vi "Main.vi"(8 "error in":errorcluster, 11 "Head Worker in":refnum<class "Head Worker.lvclass">) -> (0 "error out":errorcluster, 3 "Head Worker out":refnum<class "Head Worker.lvclass">)   [LabVIEW 2023, in "Head Worker.lvclass"]
doc: "The <b>Queued Message Handler</b> of the Worker that owns this VI."
uses:
  Head Worker.lvclass
  C:/Program Files (x86)/National Instruments/LabVIEW 2023/vi.lib/addons/_Workers/Library/Classes/Worker/Worker.lvclass
  Generated_server/RPC Service/streamai/typeDefs/Server gRPC UEs.ctl
  <vilib>/gRPC/LabVIEW gRPC Library/Server API/typeDefs/gRPCId Cluster.ctl
  <vilib>/gRPC/LabVIEW gRPC Library/Shared/grpcId.ctl
  Head Worker.lvclass/Head Worker.ctl
  Generated_server/RPC Service/streamai/streamai.lvclass
  Generated_server/RPC Service/streamai/streamai.lvclass/streamai.ctl
  rql_Start Acquisition.ctl
  rql_Stop Acquisition.ctl
  Generated_server/RPC Messages/google_protobuf_Empty.ctl
  Analog Signal/rqp_Set Signal Config.ctl
  Analog Signal/Support/Signal Config.ctl
  Analog Signal/Support/Signal Type.ctl
  Analog Signal/rqp_Set Sampling.ctl
  Analog Signal/Support/Sampling Config.ctl
  Initialization Data.ctl
  Response Cases.ctl
  <vilib>/gRPC/LabVIEW gRPC Servicer/Servicer/Servicer.lvclass
  <vilib>/gRPC/LabVIEW gRPC Servicer/ServiceBase/ServiceBase.lvclass
  Analog Signal/rqp_Insert to Subpanel.ctl
  Generated_server/RPC Messages/streamai_status.ctl
  Generated_server/RPC Messages/streamai_waveform.ctl
  Generated_server/RPC Messages/google_protobuf_Timestamp.ctl
  <vilib>/addons/_Workers/Library/Classes/Message Queue/Message Queue.lvclass
  Analog Signal/Analog Signal.lvclass
  Generated_server/Generated_server.lvlib
  <vilib>/gRPC/LabVIEW gRPC Library/grpc-lvsupport-release.lvlib
  C:/Program Files (x86)/National Instruments/LabVIEW 2023/vi.lib/addons/_Workers/Library/Classes/Workers Object/Workers Object.lvclass
  C:/Users/Admin/Documents/Learn/LabVIEW/Github_Repo/LabVIEW-Worker-gRPC/Worker gRPC Server/Workers/Head Worker/Head Worker.lvclass
panel:
  in  "Acq Status":bool
  in  "Start AI":bool
  out "Status":string
  out "Listening Port":i32
  in  "Server Address":string="localhost:50051"
  in  "Start Button":bool
  # "gRPC Server"
  # "Debug"
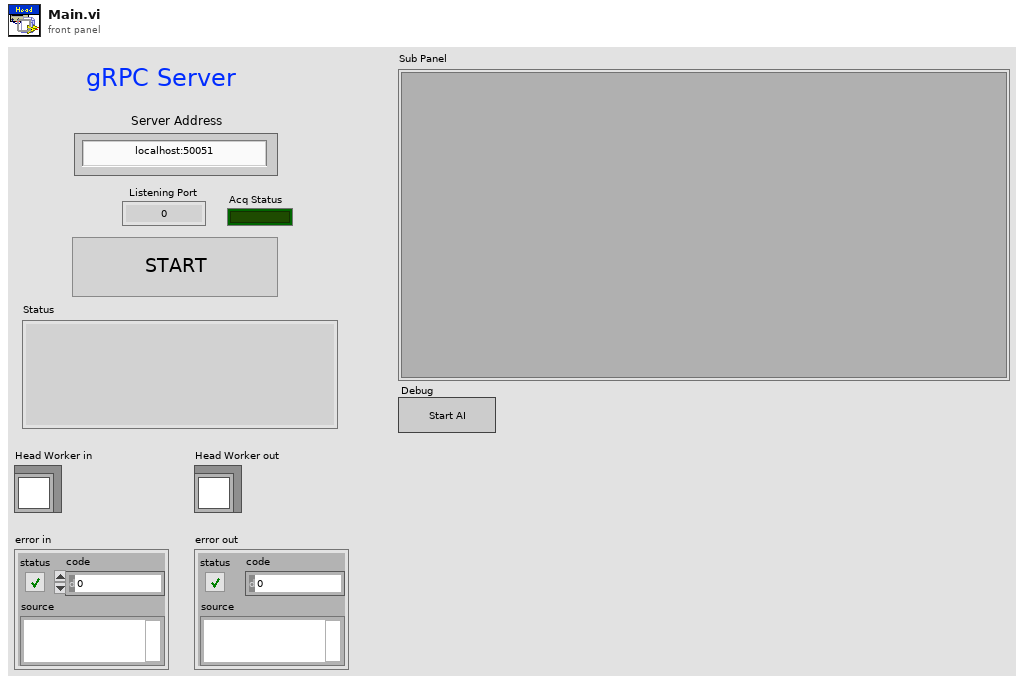
[diagram p1: front panel]
types:
  T1 = typedef "Generated_server.lvlib/streamai.lvclass/Server gRPC UEs.ctl" = cluster{"streamai startacq gRPC UE":refnum<user-event>, "streamai stopacq gRPC UE":refnum<user-event>, "streamai setSignalConfig gRPC UE":refnum<user-event>, "streamai setSamplingConfig gRPC UE":refnum<user-event>}
  T2 = typedef "Head Worker.lvclass/Event Data.ctl" = cluster{"gRPC streamAI services":refnum<user-event>, "gRPC Server Stop":refnum<user-event>}
  T3 = enum32{"Invalid", "Standard", "Closed", "Hidden", "Minimized", "Maximized"}
  T4 = typedef "Head Worker.lvclass/Initialization Data.ctl" = cluster{"Response Cases":T5}
  T5 = typedef "Head Worker.lvclass/Response Cases.ctl" = cluster{"gRPC server":refnum<class "Servicer.lvclass">, "gRPC streamAI":refnum<class "ServiceBase.lvclass">, "gRPCid Startacq":T6}
  T6 = typedef "grpc-lvsupport-release.lvlib/grpcId.ctl" = u64
  T7 = typedef "Analog Signal.lvclass/rqp_Insert to Subpanel.ctl" = cluster{"Sub Panel Ref":refnum<vi>}
  T8 = typedef "Head Worker.lvclass/rql_Start Acquisition.ctl" = cluster{"gRPCid Startacq":T6}
  T9 = typedef "Generated_server.lvlib/streamai_status.ctl" = cluster{"acquisition":bool}
  T10 = typedef "Head Worker.lvclass/rql_Stop Acquisition.ctl" = cluster{"gRPCid Stopacq":T6}
  T11 = typedef "Generated_server.lvlib/streamai_waveform.ctl" = cluster{"t0":T12, "delta_t":dbl, "values":dbl[]}
  T12 = typedef "Generated_server.lvlib/google_protobuf_Timestamp.ctl" = cluster{"seconds":i64, "nanos":i32}
  T13 = typedef "Generated_server.lvlib/google_protobuf_Empty.ctl" = cluster{"void":string}
  T14 = typedef "Analog Signal.lvclass/Signal Type.ctl" = enum16{"Sine Wave", "Square Wave"}
  T15 = typedef "Analog Signal.lvclass/rqp_Set Sampling.ctl" = cluster{"Sampling_Config":T16}
  T16 = typedef "Analog Signal.lvclass/Sampling Config.ctl" = cluster{"Fs":dbl, "#s":dbl}
  T17 = typedef "Analog Signal.lvclass/rsp_Acquisition.ctl" = cluster{"Waveform":waveform(dbl)}
  T18 = typedef "Analog Signal.lvclass/rqp_Set Signal Config.ctl" = cluster{"Signal_Config":T19, "Signal Type":T14}
  T19 = typedef "Analog Signal.lvclass/Signal Config.ctl" = cluster{"offset":dbl, "frequency":dbl, "amplitude":dbl}
  T20 = typedef "Generated_server.lvlib/streamai_signalConfig.ctl" = cluster{"type":T21, "offset":dbl, "frequency":dbl, "amplitude":dbl}
  T21 = typedef "Generated_server.lvlib/streamai_SignalType.ctl" = enum32{"SIGNAL_SINE", "SIGNAL_SQUARE"}
  T22 = typedef "Generated_server.lvlib/streamai_samplingConfig.ctl" = cluster{"sample_rate":dbl, "num_sample":i32}
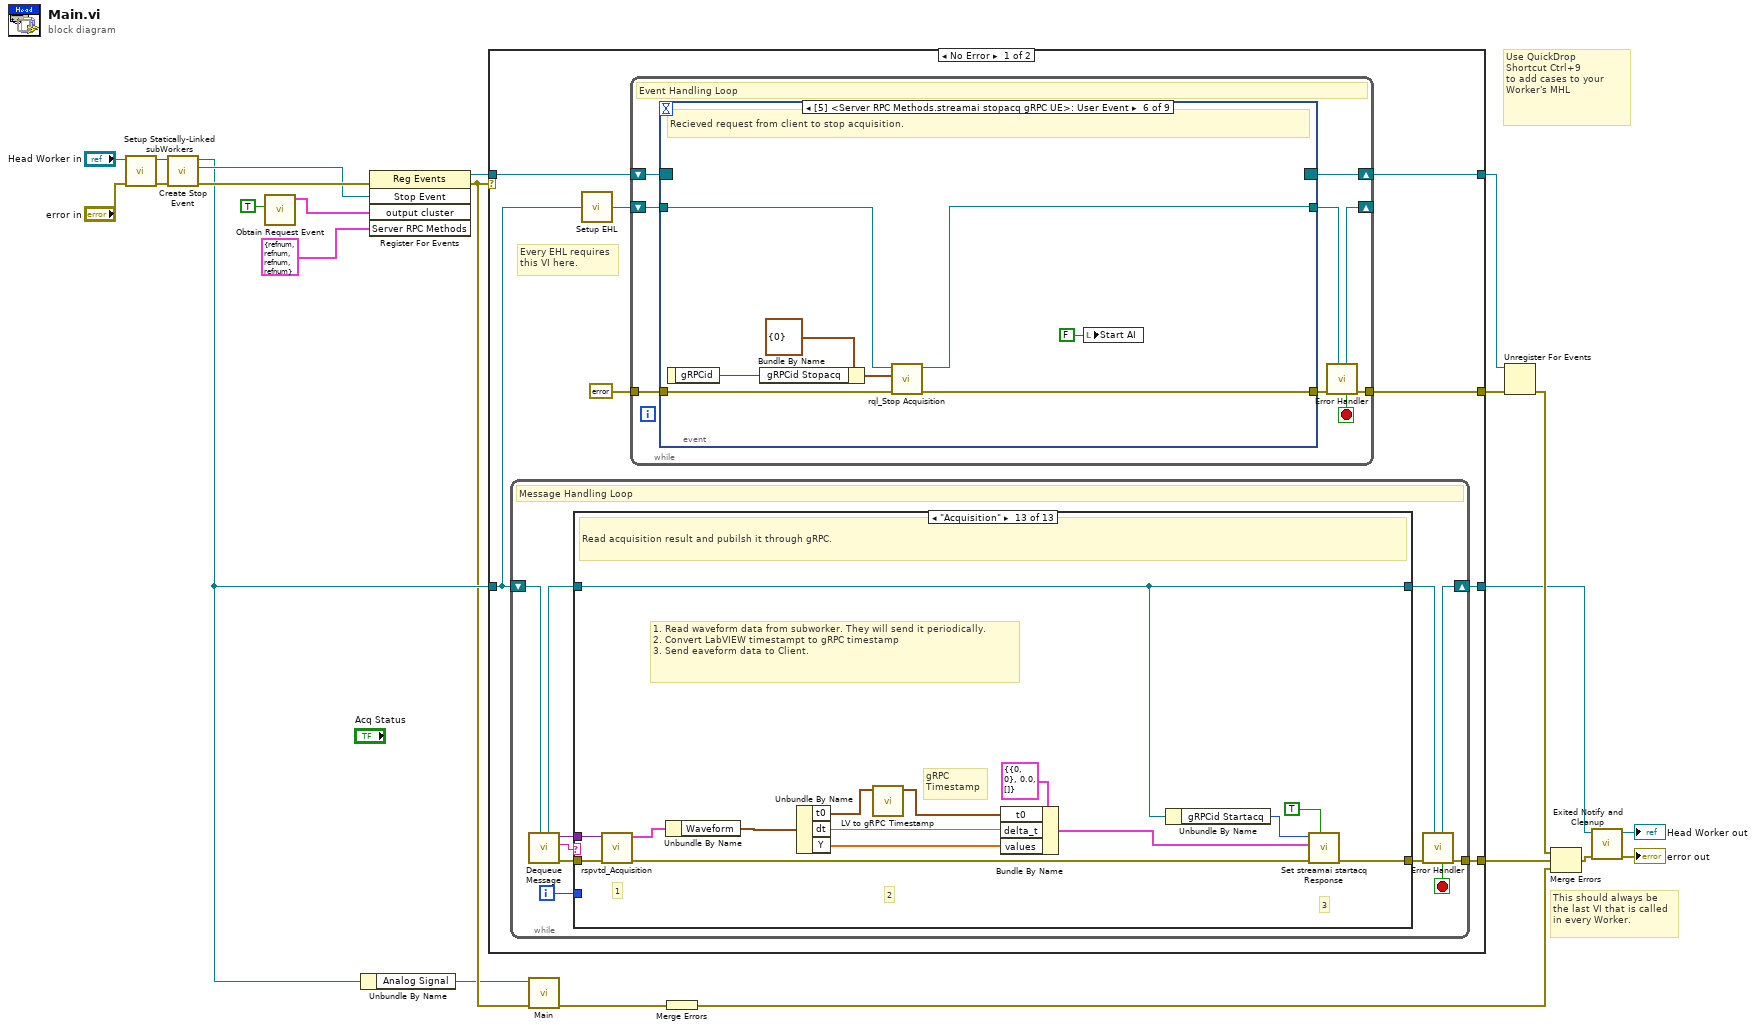
[diagram p0: block diagram]
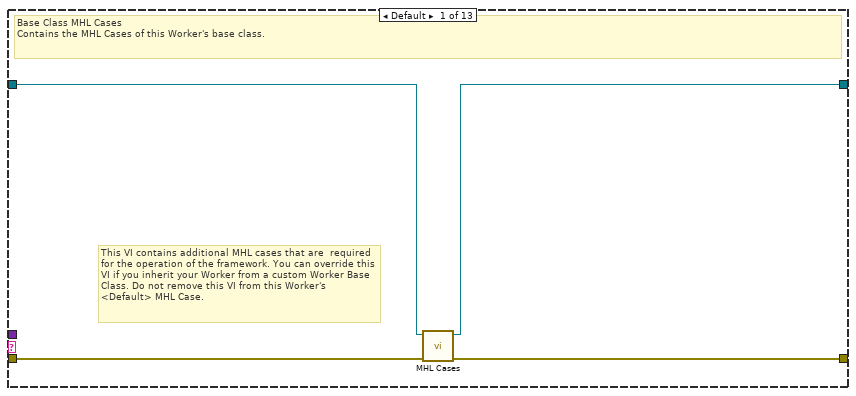
[diagram p2: hidden frame]
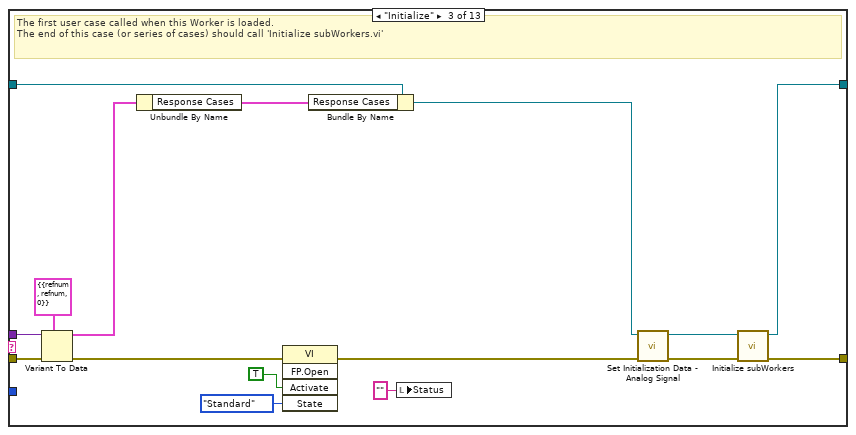
[diagram p4: hidden frame]
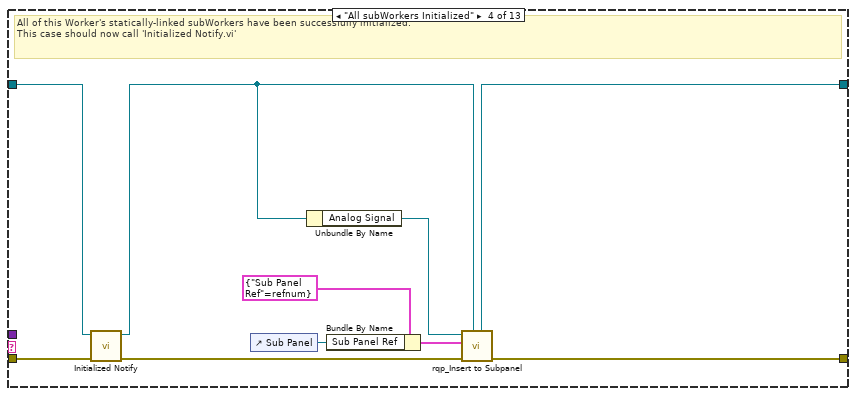
[diagram p5: hidden frame]
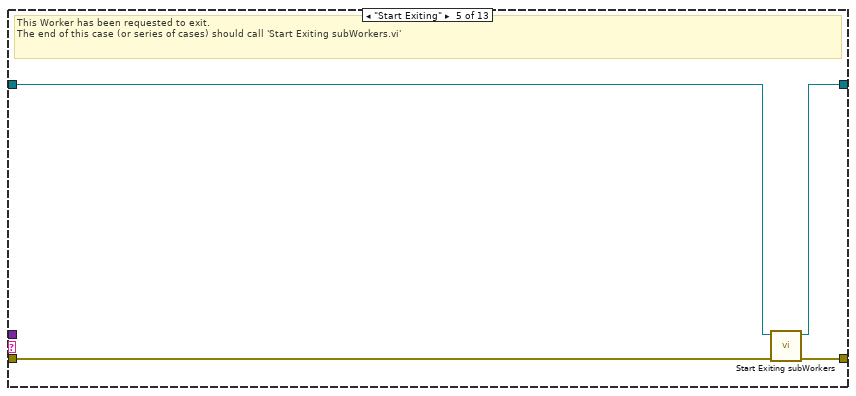
[diagram p6: hidden frame]
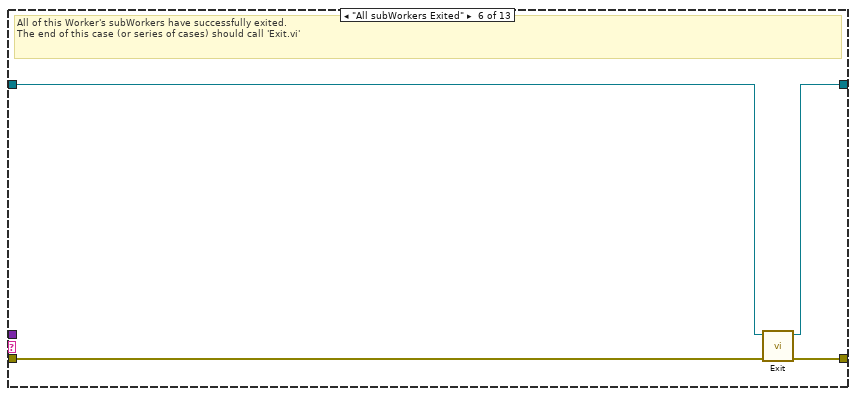
[diagram p7: hidden frame]
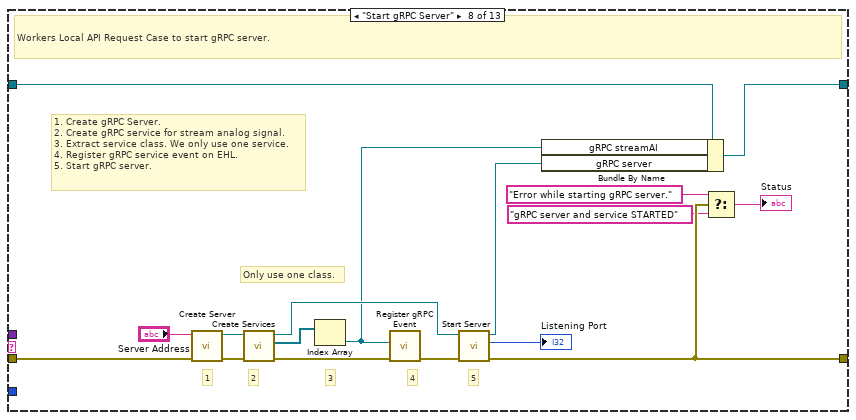
[diagram p9: hidden frame]
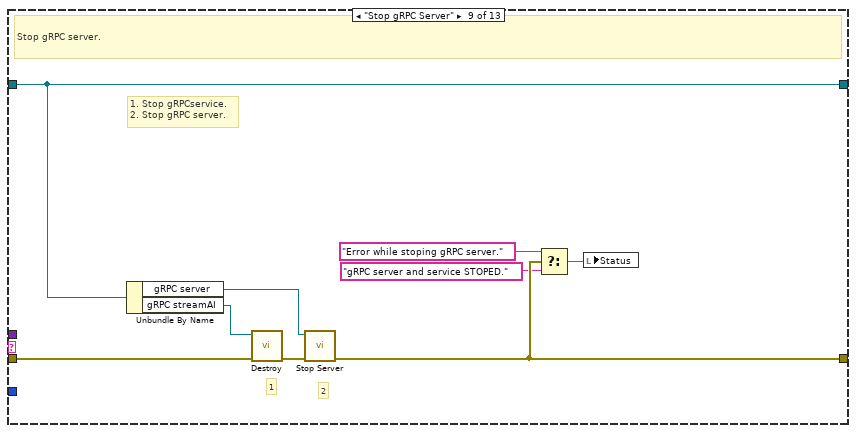
[diagram p10: hidden frame]
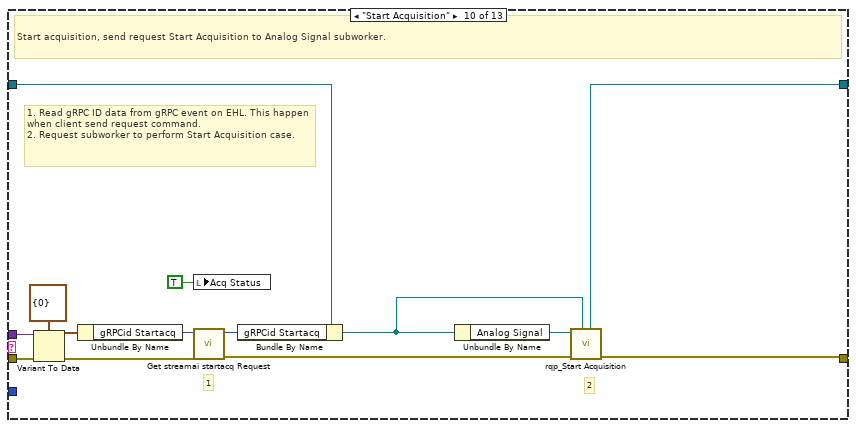
[diagram p11: hidden frame]
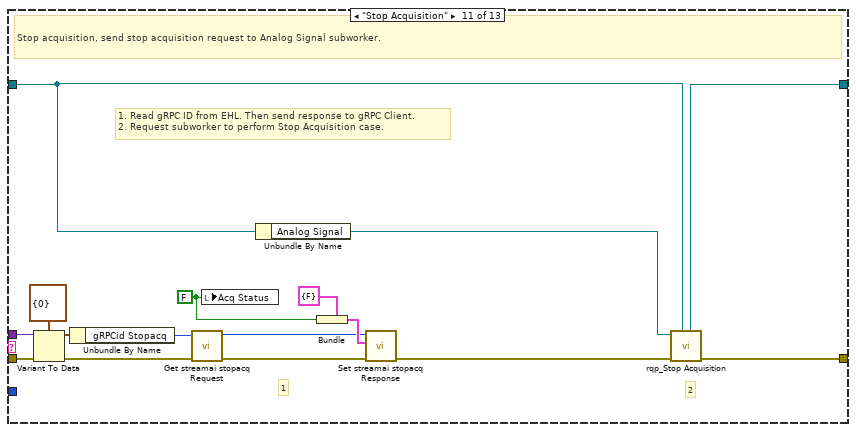
[diagram p12: hidden frame]
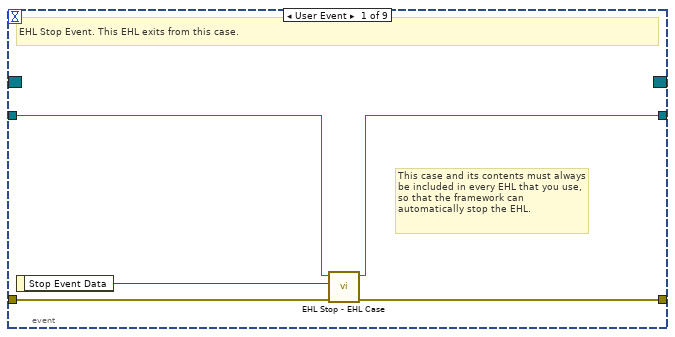
[diagram p14: hidden frame]
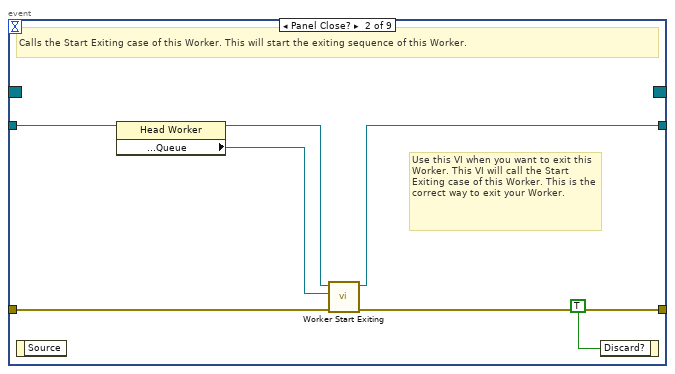
[diagram p15: hidden frame]
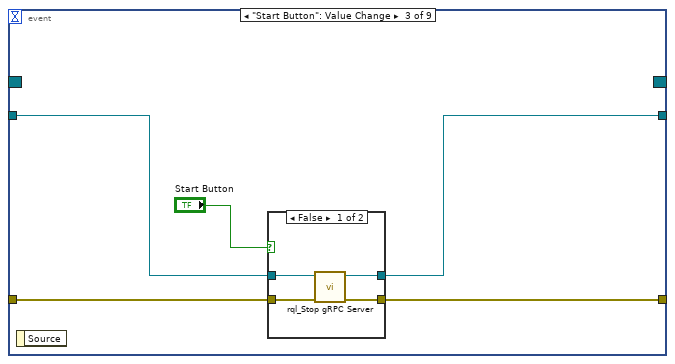
[diagram p16: hidden frame]
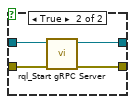
[diagram p17: hidden frame]
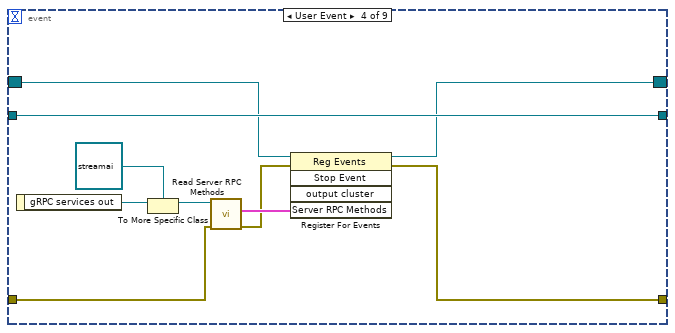
[diagram p18: hidden frame]
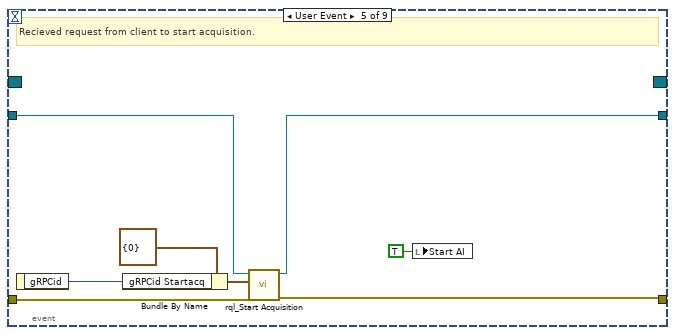
[diagram p19: hidden frame]
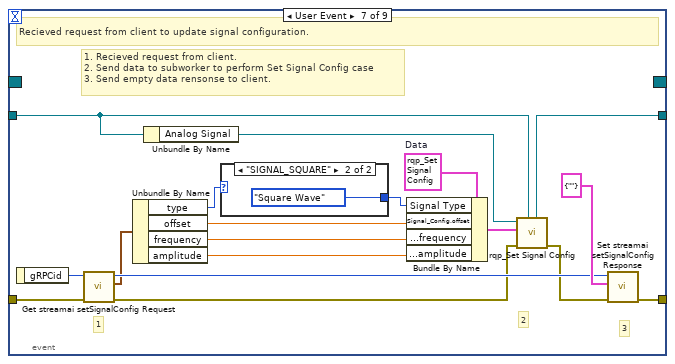
[diagram p20: hidden frame]
diagram:
  # "Use QuickDrop\nShortcut Ctrl+9\nto add cases to your\nWorker's MHL"
  # "This should always be the last VI that is called in every Worker."
  n1 = call "Setup Statically-Linked subWorkers.vi"("error in"="error in", "Head Worker in"="Head Worker in") -> ("error out"=w9:errorcluster, "Head Worker out"=w7:refnum<class "Head Worker.lvclass">)  [unwired: 8 in]
  n2 = call-dynamic "Create Stop Event.vi"("error in"=w9, "Worker"=w7) -> ("error out"=w18:errorcluster, "Stop Event"=w15:refnum<user-event>, "Worker out"=w12:refnum<class "Head Worker.lvclass">)  [unwired: 7 in]
  n3 = call "Obtain Request Event.vi"("Create New"=TRUE) -> ("output cluster"=w3:T2)  [unwired: 9 in, 1 out]
  n4 = Unbundle By Name(w12) -> ("Analog Signal"=w4:refnum<class "Analog Signal.lvclass">)
  n5 = register-events(error in=w18, w15, w3, T1 {"streamai startacq gRPC UE"=refnum, "streamai stopacq gRPC UE"=refnum, "streamai setSignalConfig gRPC UE"=refnum, "streamai setSamplingConfig gRPC UE"=refnum} ("Server RPC Methods")) -> (reference out=w17:refnum<event-registration>, error out=w10:errorcluster)  [unwired: 1 in]
  n6 = case shown="No Error" w10 {
    tunnel: w12 -> [w26 w268]
    tunnel: [w24 w269] -> w16
    tunnel: w17 -> [w31 w270]
    tunnel: [w28 w271] -> w22
    tunnel: [w30 w270] -> w21
    tunnel: [w25 w267] -> w19
    selector: w10 -> [_ w271]
    frame No Error {
      # "Every EHL requires\nthis VI here."
      n7 = while {
        shift-right: [w40] -> w25
        shift-left: w26 -> [w42]
        tunnel: [w41] -> w24
        i -> [w33]
        stop <- w34 stop-if-true
        # "Message Handling Loop"
        n8 = call-dynamic "Dequeue Message.vi"("Worker"=w42) -> ("error out"=w39:errorcluster, "Case out"=w35:string, "Data out"=w32:variant, "Worker out"=w37:refnum<class "Head Worker.lvclass">)  [unwired: 6 in, 1 out]
        n9 = case "Worker MHL Case Structure (DO NOT CHANGE LABEL NAME)" shown="\"Acquisition\"" w35 {
          tunnel: w39 -> [w46 w47 w62 w73 w75 w82 w84 w101 w110 w124 w140 w142 w157]
          tunnel: [w45 w47 w64 w71 w78 w81 w84 w98 w109 w116 w129 w142 w153] -> w38
          tunnel: w37 -> [w44 w48 w61 w74 w76 w80 w83 w100 w108 w115 w136 w141 w152]
          tunnel: [w43 w48 w63 w65 w77 w79 w83 w99 w108 w114 w135 w141 w152] -> w36
          tunnel: w33 -> [_ _ _ _ _ _ _ _ _ _ _ _ _]
          tunnel: w32 -> [_ _ w60 _ _ _ _ _ _ w122 w138 _ w155]
          frame Default {
            # "This VI contains additional MHL cases that are  required for the operation of the framework. You can override this VI if you inherit your Worker from a custom Worker Base Class. Do not remove this VI from this Worker's <Default> MHL Case."
            # "Base Class MHL Cases\nContains the MHL Cases of this Worker's base class."
            n10 = call-dynamic "MHL Cases.vi"("error in"=w46, "Worker in"=w44) -> ("error out"=w45:errorcluster, "Worker out"=w43:refnum<class "Head Worker.lvclass">)  [unwired: 8 in]
          }
          frame "------------ FRAMEWORK CASES -----------" {
            # "Start of Workers Framework Cases"
          }
          frame "Initialize" {
            # "The first user case called when this Worker is loaded.\nThe end of this case (or series of cases) should call 'Initialize subWorkers.vi'"
            n11 = Variant To Data(error in=w62, type=T4 {"Response Cases"={"gRPC server"=refnum, "gRPC streamAI"=refnum, "gRPCid Startacq"=0}} ("Initialization Data"), Variant=w60) -> (data=w59:T4, error out=w55:errorcluster)
            n12 = Unbundle By Name(w59) -> ("Response Cases"=w58:T5)
            n13 = invoke class="VI" method="FP.Open"(error in=w55, "Activate"=TRUE ("Activate?"), "State"=T3."Standard") -> (error out=w54:errorcluster)  [unwired: 2 in, 4 out]
            n14 = Bundle By Name(cluster=w61, "Response Cases"=w58) -> (w56:refnum<class "Head Worker.lvclass">)
            n15 = local write "Status"("" ("Status")) -> ()
            n16 = call "Set Initialization Data - Analog Signal.vi"("error in"=w54, "Head Worker in"=w56) -> ("error out"=w50:errorcluster, "Head Worker out"=w51:refnum<class "Head Worker.lvclass">)  [unwired: 8 in]
            n17 = call-dynamic "Initialize subWorkers.vi"("error in"=w50, "Worker"=w51) -> ("error out"=w64:errorcluster, "dup Worker out"=w63:refnum<class "Head Worker.lvclass">)  [unwired: 8 in]
          }
          frame "All subWorkers Initialized" {
            # "All of this Worker's statically-linked subWorkers have been successfully initialized.\nThis case should now call 'Initialized Notify.vi'"
            n18 = call-dynamic "Initialized Notify.vi"("error in"=w73, "Worker"=w74) -> ("error out"=w72:errorcluster, "dup Worker out"=w66:refnum<class "Head Worker.lvclass">)  [unwired: 8 in]
            n19 = control-ref of="Sub Panel"() -> (w70:refnum<vi>)
            n20 = Unbundle By Name(w66) -> ("Analog Signal"=w67:refnum<class "Analog Signal.lvclass">)
            n21 = Bundle By Name(cluster=T7 {"Sub Panel Ref"=refnum} ("Data in"), "Sub Panel Ref"=w70) -> (w68:T7)
            n22 = call "rqp_Insert to Subpanel.vi"("Caller in"=w66, "error in"=w72, "Data in"=w68, "Analog Signal in"=w67) -> ("error out"=w71:errorcluster, "dup Caller out"=w65:refnum<class "Head Worker.lvclass">)  [unwired: 5 in, 1 out]
          }
          frame "Start Exiting" {
            # "This Worker has been requested to exit. \nThe end of this case (or series of cases) should call 'Start Exiting subWorkers.vi'"
            n23 = call-dynamic "Start Exiting subWorkers.vi"("error_in"=w75, "Worker"=w76) -> ("error out"=w78:errorcluster, "dup Worker out"=w77:refnum<class "Head Worker.lvclass">)  [unwired: 8 in]
          }
          frame "All subWorkers Exited" {
            # "All of this Worker's subWorkers have successfully exited. \nThe end of this case (or series of cases) should call 'Exit.vi'"
            n24 = call-dynamic "Exit.vi"("error_in"=w82, "Worker"=w80) -> ("error out"=w81:errorcluster, "dup Worker out"=w79:refnum<class "Head Worker.lvclass">)  [unwired: 8 in]
          }
          frame "------------- LOCAL API CASES -------------" {
            # "Start of Workers Local API Cases"
          }
          frame "Start gRPC Server" {
            # "1. Create gRPC Server.\n2. Create gRPC service for stream analog signal.\n3. Extract service class. We only use one service.\n4. Register gRPC service event on EHL.\n5. Start gRPC server."
            # "5"
            # "4"
            # "3"
            # "2"
            # "1"
            # "Only use one class."
            # "Workers Local API Request Case to start gRPC server."
            n25 = call <vilib>:"Create Server.vi"("error in"=w101, "Server Address"="Server Address") -> ("error out"=w97:errorcluster, "gRPC server out"=w96:refnum<class "Servicer.lvclass">)  [unwired: 8 in]
            n26 = call "Create Services.vi"("error in (no error)"=w97, "gRPC server in"=w96) -> ("error out"=w87:errorcluster, "gRPC services out"=w88:refnum<class "ServiceBase.lvclass">[], "gRPC server out"=w94:refnum<class "Servicer.lvclass">)  [unwired: 7 in]
            n27 = Index Array(array=w88) -> (element=w85:refnum<class "ServiceBase.lvclass">)  [unwired: 1 in]
            n28 = call "Register gRPC Event.vi"("error in (no error)"=w87, "Event Data"=w85) -> ("error out"=w86:errorcluster)  [unwired: 9 in]
            n29 = call <vilib>:"Start Server.vi"("error in"=w86, "gRPC server in"=w94) -> ("error out"=w98:errorcluster, "Listening Port"=→"Listening Port":i32, "gRPC server out"=w92:refnum<class "Servicer.lvclass">)  [unwired: 7 in]
            n30 = Bundle By Name(cluster=w100, "gRPC streamAI"=w85, "gRPC server"=w92) -> (w99:refnum<class "Head Worker.lvclass">)
            n31 = Select(t="Error while starting gRPC server.", s=w98, f="gRPC server and service STARTED") -> (s? t:f=→"Status":string)
          }
          frame "Stop gRPC Server" {
            # "1. Stop gRPCservice.\n2. Stop gRPC server."
            # "2"
            # "1"
            # "Stop gRPC server."
            n32 = Unbundle By Name(w108) -> ("gRPC server"=w105:refnum<class "Servicer.lvclass">, "gRPC streamAI"=w107:refnum<class "ServiceBase.lvclass">)
            n33 = call-dynamic "Destroy.vi"("error in"=w110, "gRPC service in"=w107) -> ("error out"=w106:errorcluster)  [unwired: 8 in, 1 out]
            n34 = call <vilib>:"Stop Server.vi"("error in"=w106, "gRPC server in"=w105) -> ("error out"=w109:errorcluster)  [unwired: 9 in]
            n35 = Select(t="Error while stoping gRPC server.", s=w109, f="gRPC server and service STOPED.") -> (s? t:f=w102:string)
            n36 = local write "Status"(w102) -> ()
          }
          frame "Start Acquisition" {
            # "1. Read gRPC ID data from gRPC event on EHL. This happen when client send request command.\n2. Request subworker to perform Start Acquisition case."
            # "2"
            # "1"
            # "Start acquisition, send request Start Acquisition to Analog Signal subworker."
            n37 = Variant To Data(error in=w124, type=T8 {"gRPCid Startacq"=0} ("Data"), Variant=w122) -> (data=w121:T8, error out=w118:errorcluster)
            n38 = Unbundle By Name(w121) -> ("gRPCid Startacq"=w120:T6)
            n39 = local write "Acq Status"(TRUE ("Acq Status?")) -> ()
            n40 = call "Get streamai startacq Request.vi"("error in (no error)"=w118, "gRPCid"=w120) -> ("error out"=w117:errorcluster, "gRPCid out"=w112:T6)  [unwired: 7 in, 1 out]
            n41 = Bundle By Name(cluster=w115, "gRPCid Startacq"=w112) -> (w113:refnum<class "Head Worker.lvclass">)
            n42 = Unbundle By Name(w113) -> ("Analog Signal"=w119:refnum<class "Analog Signal.lvclass">)
            n43 = call "rqp_Start Acquisition.vi"("Caller in"=w113, "error in"=w117, "Analog Signal in"=w119) -> ("error out"=w116:errorcluster, "dup Caller out"=w114:refnum<class "Head Worker.lvclass">)  [unwired: 6 in, 1 out]
          }
          frame "Stop Acquisition" {
            w125 = FALSE ("Acq Status")
            # "1. Read gRPC ID from EHL. Then send response to gRPC Client.\n2. Request subworker to perform Stop Acquisition case."
            # "2"
            # "1"
            # "Stop acquisition, send stop acquisition request to Analog Signal subworker."
            n44 = Variant To Data(error in=w140, type=T10 {"gRPCid Stopacq"=0} ("Data"), Variant=w138) -> (data=w128:T10, error out=w131:errorcluster)
            n45 = Unbundle By Name(w128) -> ("gRPCid Stopacq"=w127:T6)
            n46 = call "Get streamai stopacq Request.vi"("error in (no error)"=w131, "gRPCid"=w127) -> ("error out"=w130:errorcluster, "gRPCid out"=w133:T6)  [unwired: 7 in, 1 out]
            n47 = local write "Acq Status"(w125) -> ()
            n48 = Unbundle By Name(w136) -> ("Analog Signal"=w137:refnum<class "Analog Signal.lvclass">)
            n49 = Bundle(cluster=T9 {"acquisition"=FALSE} ("Message Data"), "acquisition"=w125) -> (w134:T9)
            n50 = call "Set streamai stopacq Response.vi"("error in (no error)"=w130, "Message Data"=w134, "gRPCid in"=w133) -> ("error out"=w126:errorcluster)  [unwired: 8 in]
            n51 = call "rqp_Stop Acquisition.vi"("Caller in"=w136, "error in"=w126, "Analog Signal in"=w137) -> ("error out"=w129:errorcluster, "dup Caller out"=w135:refnum<class "Head Worker.lvclass">)  [unwired: 6 in, 1 out]
          }
          frame "------------- RESPONSE CASES --------------" {
            # "Start of Workers Response Cases"
          }
          frame "Acquisition" {
            # "3"
            # "2"
            # "1"
            # "1. Read waveform data from subworker. They will send it periodically.\n2. Convert LabVIEW timestampt to gRPC timestamp\n3. Send eaveform data to Client."
            # "gRPC\nTimestamp"
            # "Read acquisition result and pubilsh it through gRPC."
            n52 = call "rspvtd_Acquisition.vi"("error in"=w157, "Data in"=w155) -> ("error out"=w156:errorcluster, "Data out"=w154:T17)  [unwired: 8 in]
            n53 = Unbundle By Name(w154) -> ("Waveform"=w148:waveform(dbl))
            n54 = Unbundle By Name(w148) -> ("t0"=w144:timestamp, "dt"=w146:dbl, "Y"=w147:dbl[])
            n55 = call "LV to gRPC Timestamp.vi"("LV Timestamp"=w144) -> ("gRPC Timestamp"=w143:T12)  [unwired: 10 in]
            n56 = Bundle By Name(cluster=T11 {"t0"={"seconds"=0, "nanos"=0}, "delta_t"=0.0, "values"=[]} ("Message Data"), "t0"=w143, "delta_t"=w146, "values"=w147) -> (w145:T11)
            n57 = Unbundle By Name(w152) -> ("gRPCid Startacq"=w151:T6)
            n58 = call "Set streamai startacq Response.vi"("Streaming? (F)"=TRUE, "error in (no error)"=w156, "Message Data"=w145, "gRPCid in"=w151) -> ("error out"=w153:errorcluster)  [unwired: 7 in]
          }
        }
        n59 = call-dynamic "Error Handler.vi"("Worker"=w36, "error_in"=w38) -> ("error out"=w41:errorcluster, "Stop Loop"=w34:bool, "Worker out"=w40:refnum<class "Head Worker.lvclass">)  [unwired: 7 in]
      }
      n60 = call-dynamic "Setup EHL.vi"("Worker"=w26) -> ("Worker out"=w27:refnum<class "Head Worker.lvclass">)  [unwired: 14 in]
      n61 = while "Event Handling Loop" {
        shift-right: [w166] -> w30
        shift-left: w31 -> [w165]
        tunnel: [w161] -> w28
        tunnel: errorcluster {"status"=FALSE, "code"=0, "source"=""} ("error constant") -> [w163]
        shift-right: [w159] -> _
        shift-left: w27 -> [w164]
        stop <- w158 stop-if-true
        # "Event Handling Loop"
        n62 = event shown="[5] <Server RPC Methods.streamai stopacq gRPC UE>: User Event" {
          selector: w165 -> [_ _ _ w200 _ _ _ _ _]
          dyn-events: [_ _ _ w199 _ _ _ _ _] -> w166
          timeout: _ -> [_ _ _ _ _ _ _ _ _]
          tunnel: [w170 w177 w182 w192 w205 w216 w233 w246 w255] -> w162
          tunnel: w163 -> [w171 w176 w183 w194 w206 w217 w234 w249 w256]
          tunnel: w164 -> [w169 w175 w181 w201 w204 w212 w219 w239 w252]
          tunnel: [w168 w174 w180 w201 w203 w211 w218 w238 w254] -> w160
          event User Event {
            # "This case and its contents must always be included in every EHL that you use, so that the framework can automatically stop the EHL."
            # "EHL Stop Event. This EHL exits from this case."
            n63 = event-data() -> ("Stop Event Data"=w167:variant)  [unwired: 1 in]
            n64 = call-dynamic "EHL Stop - EHL Case.vi"("error in"=w171, "Stop Event Data"=w167, "Worker"=w169) -> ("error out"=w170:errorcluster, "Worker out"=w168:refnum<class "Head Worker.lvclass">)  [unwired: 7 in]
          }
          event Panel Close? {
            # "Use this VI when you want to exit this Worker. This VI will call the Start Exiting case of this Worker. This is the correct way to exit your Worker."
            # "Calls the Start Exiting case of this Worker. This will start the exiting sequence of this Worker."
            n65 = event-data() -> ()  [unwired: 1 in, 1 out]
            n66 = property class="Head Worker"(reference=w175) -> (reference out=w173:refnum<class "Head Worker.lvclass">, "Accessors:Read:Public API:Queue"=w172:refnum<class "Message Queue.lvclass">)  [unwired: 1 in, 1 out]
            n67 = call-dynamic "Worker Start Exiting.vi"("error_in"=w176, "Message Queue"=w172, "Worker"=w173) -> ("error out"=w177:errorcluster, "dup Worker out"=w174:refnum<class "Head Worker.lvclass">)  [unwired: 7 in]
            n68 = event-data ("Event Filter Node")("Discard?"=TRUE) -> ()  [unwired: 1 in, 1 out]
          }
          event "Start Button": Value Change {
            n69 = event-data() -> ()  [unwired: 1 in, 1 out]
            n70 = case shown="False" "Start Button" {
              tunnel: w183 -> [w187 w191]
              tunnel: [w186 w190] -> w182
              tunnel: w181 -> [w184 w189]
              tunnel: [w185 w188] -> w180
              frame False {
                n71 = call "rql_Stop gRPC Server.vi"("error in"=w187, "Head Worker in"=w184) -> ("error out"=w186:errorcluster, "dup Head Worker out"=w185:refnum<class "Head Worker.lvclass">)  [unwired: 8 in]
              }
              frame True {
                n72 = call "rql_Start gRPC Server.vi"("error in"=w191, "Head Worker in"=w189) -> ("error out"=w190:errorcluster, "dup Head Worker out"=w188:refnum<class "Head Worker.lvclass">)  [unwired: 8 in]
              }
            }
          }
          event User Event {
            n73 = event-data() -> ("gRPC services out"=w198:refnum<class "ServiceBase.lvclass">)  [unwired: 1 in]
            n74 = To More Specific Class(target class=refnum<class "streamai.lvclass"> refnum ("gRPC service in"), reference=w198) -> (specific class reference=w196:refnum<class "streamai.lvclass">)  [unwired: 1 in, 1 out]
            n75 = call "Read Server RPC Methods.vi"("error in (no error)"=w194, "gRPC service in"=w196) -> ("error out"=w193:errorcluster, "Server RPC Methods"=w195:T1)  [unwired: 7 in, 1 out]
            n76 = register-events(reference=w200, error in=w193, w195) -> (reference out=w199:refnum<event-registration>, error out=w192:errorcluster)  [unwired: 2 in]
          }
          event User Event {
            # "Recieved request from client to start acquisition."
            n77 = event-data() -> ("gRPCid"=w208:T6)  [unwired: 1 in]
            n78 = Bundle By Name(cluster=T8 {"gRPCid Startacq"=0} ("Data in"), "gRPCid Startacq"=w208) -> (w207:T8)
            n79 = call "rql_Start Acquisition.vi"("error in"=w206, "Data in"=w207, "Head Worker in"=w204) -> ("error out"=w205:errorcluster, "dup Head Worker out"=w203:refnum<class "Head Worker.lvclass">)  [unwired: 7 in]
            n80 = local write "Start AI"(TRUE ("Start AI")) -> ()
          }
          event User Event {
            # "Recieved request from client to stop acquisition."
            n81 = event-data() -> ("gRPCid"=w215:T6)  [unwired: 1 in]
            n82 = Bundle By Name(cluster=T10 {"gRPCid Stopacq"=0} ("Data"), "gRPCid Stopacq"=w215) -> (w213:T10)
            n83 = call "rql_Stop Acquisition.vi"("error in"=w217, "Data in"=w213, "Head Worker in"=w212) -> ("error out"=w216:errorcluster, "dup Head Worker out"=w211:refnum<class "Head Worker.lvclass">)  [unwired: 7 in]
            n84 = local write "Start AI"(FALSE ("Start AI")) -> ()
          }
          event User Event {
            w229 = T18 {"Signal_Config"={"offset"=0.0, "frequency"=10.0, "amplitude"=1.0}, "Signal Type"=enum."Sine Wave"}  # Data
            # "3"
            # "2"
            # "1"
            # "1. Recieved request from client.\n2. Send data to subworker to perform Set Signal Config case\n3. Send empty data rensonse to client."
            # "Recieved request from client to update signal configuration."
            n85 = event-data() -> ("gRPCid"=w235:T6)  [unwired: 1 in]
            n86 = call "Get streamai setSignalConfig Request.vi"("error in (no error)"=w234, "gRPCid"=w235) -> ("error out"=w223:errorcluster, "Message Data"=w230:T20, "gRPCid out"=w231:T6)  [unwired: 7 in]
            n87 = Unbundle By Name(w230) -> ("type"=w225:T21, "offset"=w228:dbl, "frequency"=w227:dbl, "amplitude"=w226:dbl)
            n88 = Unbundle By Name(w219) -> ("Analog Signal"=w220:refnum<class "Analog Signal.lvclass">)
            n89 = case shown="\"SIGNAL_SQUARE\"" w225 {
              tunnel: [Signal_Type."Sine Wave" ("Signal Type") Signal_Type."Square Wave" ("Signal Type")] -> w224
              frame "SIGNAL_SINE", Default {
              }
              frame "SIGNAL_SQUARE" {
              }
            }
            n90 = Bundle By Name(cluster=w229, "Signal Type"=w224, "Signal_Config.offset"=w228, "Signal_Config.frequency"=w227, "Signal_Config.amplitude"=w226) -> (w221:T18)
            n91 = call "rqp_Set Signal Config.vi"("Caller in"=w219, "error in"=w223, "Data in"=w221, "Analog Signal in"=w220) -> ("error out"=w222:errorcluster, "dup Caller out"=w218:refnum<class "Head Worker.lvclass">)  [unwired: 5 in, 1 out]
            n92 = call "Set streamai setSignalConfig Response.vi"("error in (no error)"=w222, "Message Data"=T13 {"void"=""}, "gRPCid in"=w231) -> ("error out"=w233:errorcluster)  [unwired: 8 in]
          }
          event User Event {
            # "3"
            # "2"
            # "1"
            # "1. Recieved request from client.\n2. Send data to subworker to perform Set Sampling case\n3. Send empty data rensonse to client."
            # "Recieved request from client to update acquisition sampling configuration."
            n93 = event-data() -> ("gRPCid"=w250:T6)  [unwired: 1 in]
            n94 = Unbundle By Name(w239) -> ("Analog Signal"=w243:refnum<class "Analog Signal.lvclass">)
            n95 = call "Get streamai setSamplingConfig Request.vi"("error in (no error)"=w249, "gRPCid"=w250) -> ("error out"=w241:errorcluster, "Message Data"=w244:T22, "gRPCid out"=w248:T6)  [unwired: 7 in]
            n96 = Bundle By Name(cluster=T15 {"Sampling_Config"={"Fs"=1000.0, "#s"=1000.0}} ("Data"), "Sampling_Config"=w244) -> (w242:T15)
            n97 = call "rqp_Set Sampling.vi"("Caller in"=w239, "error in"=w241, "Data in"=w242, "Analog Signal in"=w243) -> ("error out"=w240:errorcluster, "dup Caller out"=w238:refnum<class "Head Worker.lvclass">)  [unwired: 5 in, 1 out]
            n98 = call "Set streamai setSamplingConfig Response.vi"("error in (no error)"=w240, "Message Data"=T13 {"void"=""}, "gRPCid in"=w248) -> ("error out"=w246:errorcluster)  [unwired: 8 in]
          }
          event "Start AI": Value Change {
            # "Only for debug."
            n99 = event-data() -> ()  [unwired: 1 in, 1 out]
            n100 = Unbundle By Name(w252) -> ("Analog Signal"=w251:refnum<class "Analog Signal.lvclass">)
            n101 = case shown="False" "Start AI" {
              tunnel: w256 -> [w261 w266]
              tunnel: [w260 w265] -> w255
              tunnel: w252 -> [w259 w263]
              tunnel: [w258 w264] -> w254
              tunnel: w251 -> [w257 w262]
              frame False {
                n102 = call "rqp_Stop Acquisition.vi"("Caller in"=w259, "error in"=w261, "Analog Signal in"=w257) -> ("error out"=w260:errorcluster, "dup Caller out"=w258:refnum<class "Head Worker.lvclass">)  [unwired: 6 in, 1 out]
              }
              frame True {
                n103 = call "rqp_Start Acquisition.vi"("Caller in"=w263, "error in"=w266, "Analog Signal in"=w262) -> ("error out"=w265:errorcluster, "dup Caller out"=w264:refnum<class "Head Worker.lvclass">)  [unwired: 6 in, 1 out]
              }
            }
          }
        }
        n104 = call-dynamic "Error Handler.vi"("Worker"=w160, "error_in"=w162) -> ("error out"=w161:errorcluster, "Stop Loop"=w158:bool, "Worker out"=w159:refnum<class "Head Worker.lvclass">)  [unwired: 7 in]
      }
    }
    frame Error {
      n105 = call-dynamic "Error Handler.vi"("Worker"=w268, "error_in"=w271) -> ("error out"=w269:errorcluster, "Worker out"=w267:refnum<class "Head Worker.lvclass">)  [unwired: 7 in, 1 out]
    }
  }
  n106 = call-dynamic "Main.vi"("error in"=w10, "Analog Signal in"=w4) -> ("error out"=w5:errorcluster)  [unwired: 8 in, 1 out]
  n107 = Merge Errors(w5) -> (w6:errorcluster)
  n108 = Unregister For Events(event registration refnum=w21, error in=w22) -> (error out=w23:errorcluster)
  n109 = Merge Errors(w23, w16, w6) -> (w20:errorcluster)
  n110 = call-dynamic "Exited Notify and Cleanup.vi"("error_in"=w20, "Worker"=w19) -> ("error out"=→"error out":errorcluster, "dup Worker out"=→"Head Worker out":refnum<class "Head Worker.lvclass">)  [unwired: 8 in]
